vi "Cancel_Query.vi"(8 "error in (no error)":errorcluster, 11 "Postgres Connector In":refnum<class "Postgres Connector.lvclass">) -> (0 "error out":errorcluster)   [LabVIEW 2020, in "Postgres Connector.lvclass"]
doc: "This VI is used to cancel a query. It open a TCP connection and cancel the actual query. There is no need to close the connection after because the server will close it automatically.\ns"
uses:
  Postgres Connector.lvclass
  Postgres Connector.lvclass/Postgres Connector.ctl
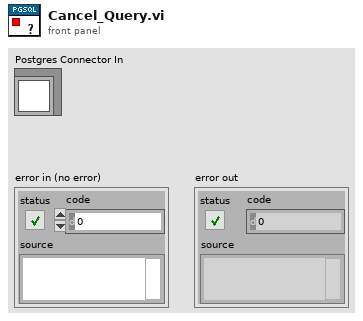
[diagram p1: front panel]
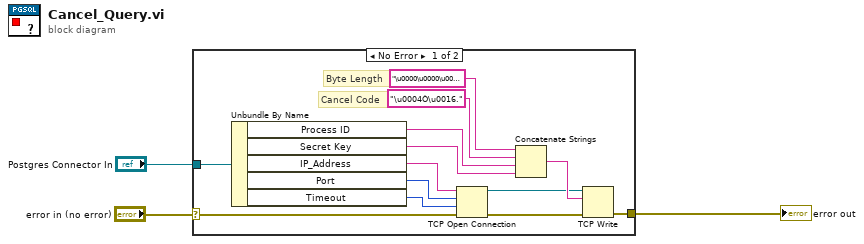
[diagram p0: block diagram]
diagram:
  n1 = case shown="No Error" "error in (no error)" {
    selector: "error in (no error)" -> [w6 w17]
    tunnel: "Postgres Connector In" -> [w9 _]
    tunnel: [w7 w17] -> w3
    frame No Error {
      # "Cancel Code"
      # "Byte Length"
      n2 = Unbundle By Name(w9) -> ("Process ID"=w5:string, "Secret Key"=w4:string, "IP_Address"=w16:string, "Port"=w15:u16, "Timeout"=w14:i32)
      n3 = TCP Open Connection(address=w16, remote port or service name=w15, timeout ms (60000)=w14, error in (no error)=w6) -> (connection ID=w8:refnum<k5>, error out=w13:errorcluster)  [unwired: 1 in]
      n4 = Concatenate Strings("\u0000\u0000\u0000\u0010", "\u0004Ò\u0016." ("string"), w5, w4) -> (w10:string)
      n5 = TCP Write(connection ID=w8, data in=w10, error in (no error)=w13) -> (error out=w7:errorcluster)  [unwired: 1 in, 2 out]
    }
    frame Error {
    }
  }
  "error out" <- w3
